vi "Close File.vi"(8 "error in (no error)":errorcluster, 11 "TIFF in":refnum<class "TIFF.lvclass">) -> (0 "error out":errorcluster, 3 "TIFF out":refnum<class "TIFF.lvclass">)   [LabVIEW 2018, in "BinaryTIFF.lvlib" / "TIFF.lvclass"]
uses:
  TIFF.lvclass
  TIFF.lvclass/TIFF.ctl
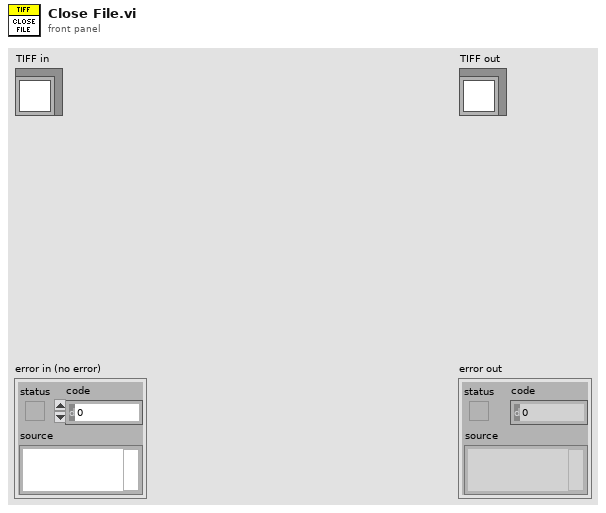
[diagram p1: front panel]
types:
  T1 = enum16{"<not opened>", "Open for Read", "Open for Write"}
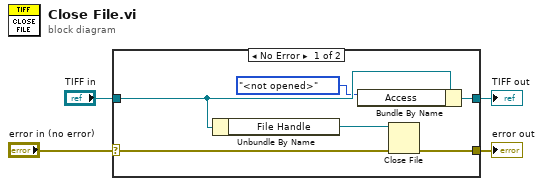
[diagram p0: block diagram]
diagram:
  n1 = case shown="No Error" "error in (no error)" {
    selector: "error in (no error)" -> [w6 w11]
    tunnel: [w5 w11] -> w4
    tunnel: "TIFF in" -> [w9 w12]
    tunnel: [w7 w12] -> w2
    frame No Error {
      n2 = Unbundle By Name(w9) -> ("File Handle"=w10:refnum<file>)
      n3 = Bundle By Name(cluster=w9, "Access"=T1."<not opened>" ("File Info.Access")) -> (w7:refnum<class "TIFF.lvclass">)
      n4 = Close File(refnum=w10, error in=w6) -> (error out=w5:errorcluster)  [unwired: 1 out]
    }
    frame Error {
    }
  }
  "error out" <- w4
  "TIFF out" <- w2
